vi "Broadcast Event.vi"(6 "error in (no error)":errorcluster, 7 "Event Data":refnum<class "Event.lvclass">, 8 "View Enqueuer":refnum<class "Message Enqueuer.lvclass">, 9 "Controller Actor in":refnum<class "Controller Actor.lvclass">) -> (0 "error out":errorcluster)   [LabVIEW 2016, in "Event Actors.lvlib" / "Controller Actor.lvclass"]
uses:
  Controller Actor.lvclass
  Event/Event.lvclass
  <vilib>/ActorFramework/Message Enqueuer/Message Enqueuer.lvclass
  Controller Actor.lvclass/Controller Actor.ctl
  Event Handler Details.ctl
  Event Handlers/Event Generated Msg/Event Generated Msg.lvclass
  C:/Program Files (x86)/National Instruments/LabVIEW 2016/vi.lib/ActorFramework/Message/Message.lvclass
  Event Handlers/Event Generated Msg/Event Generated Msg.lvclass/Event Generated Msg.ctl
  <vilib>/ActorFramework/Message Enqueuer/Message Enqueuer.lvclass/Message Enqueuer.ctl
  <vilib>/ActorFramework/Message Enqueuer/Enqueue.vi
  <vilib>/Utility/LVClass/Get LV Class Name.vi
  <resource>/AFDebug/Generate Trace for Message.vi
  <vilib>/ActorFramework/Message Priority Queue/Priority Enqueue.vi
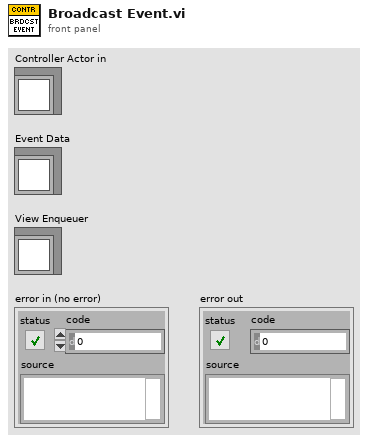
[diagram p1: front panel]
types:
  T1 = typedef "Event Actors.lvlib/Controller Actor.lvclass/Event Handler Details.ctl" = cluster{"Exclude From Broadcast":bool, "Paused":bool, "View Event Fire Handler":refnum<class "Event Generated Msg.lvclass">}
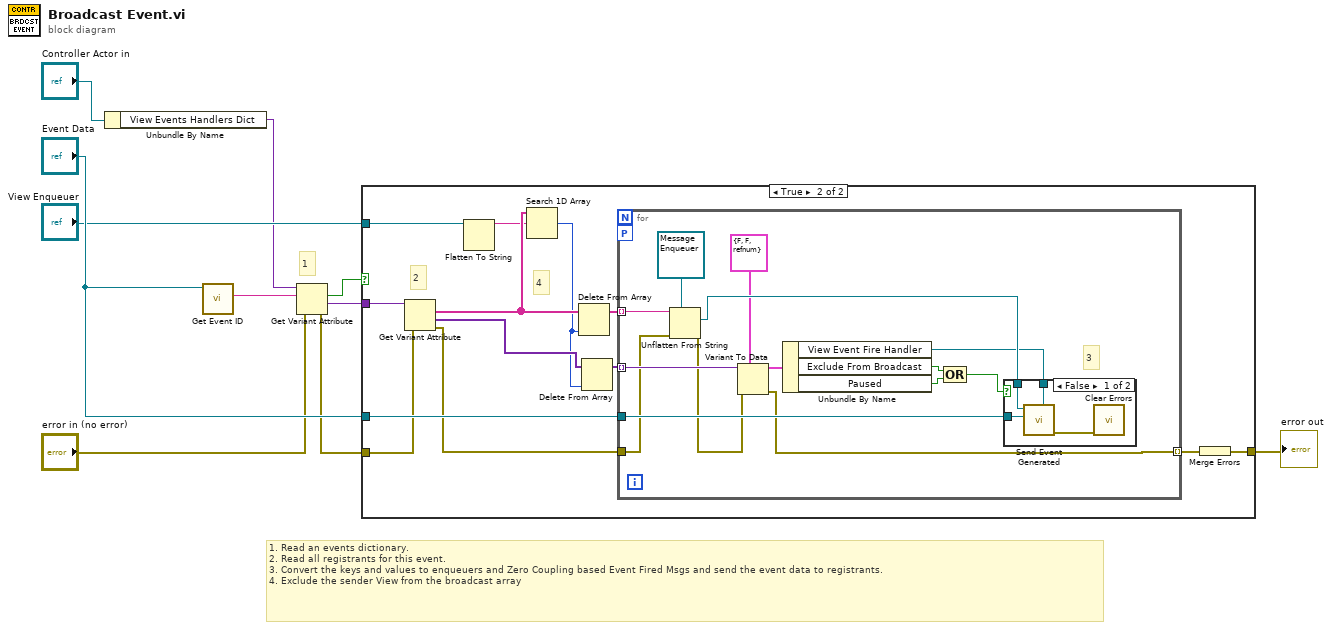
[diagram p0: block diagram]
diagram:
  # "1. Read an events dictionary.\n2. Read all registrants for this event.\n3. Convert the keys and values to enqueuers and Zero Coupling based Event Fired Msgs and send the event data to registrants.\n4. Exclude the sender View from the broadcast array"
  # "1"
  n1 = Unbundle By Name("Controller Actor in") -> ("View Events Handlers Dict"=w1:variant)
  n2 = call-dynamic "Get Event ID.vi"("Event in"="Event Data") -> ("Event ID"=w5:string)  [unwired: 8 in, 2 out]
  n3 = Get Variant Attribute(Variant=w1, name=w5, error in="error in (no error)") -> (found=w4:bool, value=w3:variant, error out=w2:errorcluster)  [unwired: 1 in, 1 out]
  n4 = case shown="True" w4 {
    tunnel: w3 -> [_ w22]
    tunnel: "Event Data" -> [_ w24]
    tunnel: w2 -> [w11 w21]
    tunnel: [w11 w12] -> w8
    tunnel: "View Enqueuer" -> [_ w17]
    frame False {
    }
    frame True {
      # "4"
      # "2"
      n5 = Get Variant Attribute(Variant=w22, error in=w21) -> (names=w19:string[], values=w15:variant[], error out=w20:errorcluster)  [unwired: 2 in, 1 out]
      n6 = Flatten To String(anything=w17) -> (data string=w16:string)  [unwired: 3 in, 2 out]
      n7 = Search 1D Array(1D array=w19, element=w16) -> (index of element=w13:i32)  [unwired: 1 in]
      n8 = Delete From Array(array=w19, index=w13) -> (array with subset deleted=w18:string[])  [unwired: 1 in, 1 out]
      n9 = Delete From Array(array=w15, index=w13) -> (array with subset deleted=w14:variant[])  [unwired: 1 in, 1 out]
      n10 = for {
        tunnel: w18 -> [w38] mode=indexing
        tunnel: w14 -> [w37] mode=indexing
        tunnel: w24 -> [w34]
        tunnel: w20 -> [w33]
        tunnel: [w29] -> w23 mode=indexing
        workers-P: _ -> [_]
        # "3"
        n11 = Unflatten From String(type=refnum<class "Message Enqueuer.lvclass"> refnum ("Message Enqueuer"), binary string=w38, error in (no error)=w33) -> (value=w36:refnum<class "Message Enqueuer.lvclass">, error out=w32:errorcluster)  [unwired: 2 in, 1 out]
        n12 = Variant To Data(error in=w32, type=T1 {"Exclude From Broadcast"=FALSE, "Paused"=FALSE, "View Event Fire Handler"=refnum} ("Message Type"), Variant=w37) -> (data=w35:T1, error out=w29:errorcluster)
        n13 = Unbundle By Name(w35) -> ("View Event Fire Handler"=w27:refnum<class "Event Generated Msg.lvclass">, "Exclude From Broadcast"=w26:bool, "Paused"=w25:bool)
        n14 = Compound Arithmetic op=OR(w26, w25) -> (w28:bool)
        n15 = case shown="False" w28 {
          tunnel: w27 -> [w42 _]
          tunnel: w34 -> [w41 _]
          tunnel: w36 -> [w39 _]
          frame False {
            n16 = call "Send Event Generated.vi"("Message Type"=w42, "Event Data"=w41, "Message Enqueuer"=w39) -> ("Error Out"=w40:errorcluster)  [unwired: 7 in, 1 out]
            n17 = call <vilib>:"Clear Errors.vi"("error in (no error)"=w40) -> ()  [unwired: 5 in, 2 out]
          }
          frame True {
          }
        }
      }
      n18 = Merge Errors(w23) -> (w12:errorcluster)
    }
  }
  "error out" <- w8
